vi "Read.vi"(8 "error in (no error)":errorcluster, 11 "Const_WFM in":refnum<class "Const_WFM_1D.lvclass">) -> (0 "error out":errorcluster, 2 "Waveform":waveform(dbl)[](array[waveform]), 3 "Const_WFM out":refnum<class "Const_WFM_1D.lvclass">)   [LabVIEW 2021, in "Const_WFM_1D.lvclass"]
uses:
  Const_WFM_1D.lvclass
  Const_WFM_1D.lvclass/Const_WFM_1D.ctl
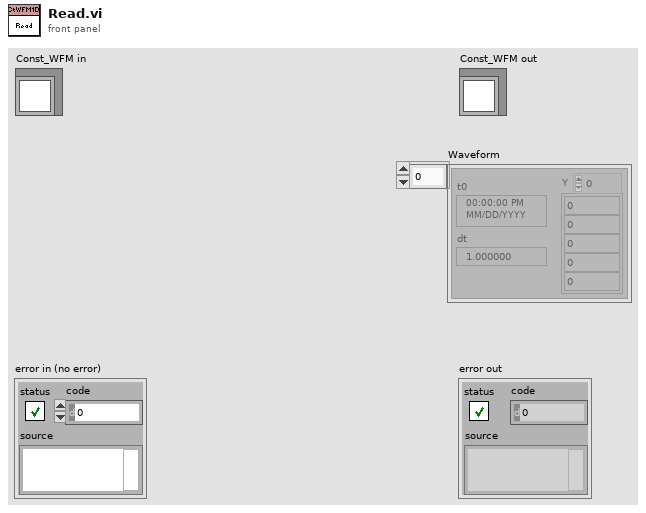
[diagram p1: front panel]
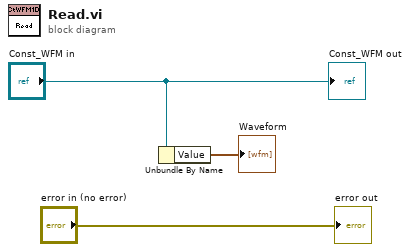
[diagram p0: block diagram]
diagram:
  n1 = Unbundle By Name("Const_WFM in") -> ("Value"=→"Waveform":waveform(dbl)[])
  "error out" <- "error in (no error)"
  "Const_WFM out" <- "Const_WFM in"
